vi "CRYInit Data & result stacks global.vi"(8 "Set Value":bool, 9 "No Project Exist?":bool=TRUE, 10 "Pause Proc":bool, 11 "Init?":bool) -> ()   [LabVIEW 2013]
uses:
  CRYData & result stacks global.vi
  CRYWindow/SubVI/CRYMain Sub Window Global.vi
panel:
  # "Set Toolbar Time, Lot, S/N, Iteration value."
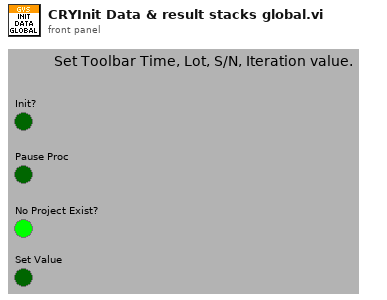
[diagram p1: front panel]
types:
  T1 = enum8{"Enabled", "Disabled", "Disabled and Grayed Out"}
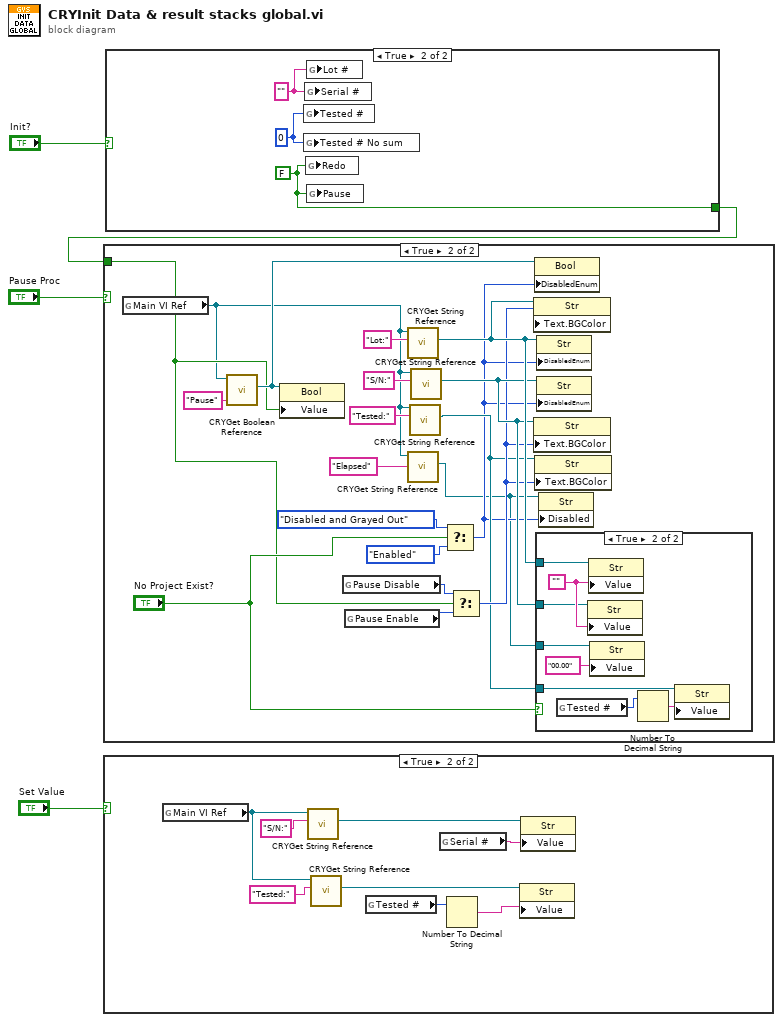
[diagram p0: block diagram]
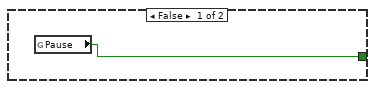
[diagram p3: hidden frame]
diagram:
  n1 = case shown="True" "Set Value" {
    frame False {
    }
    frame True {
      n2 = global read "CRYMain Sub Window Global.vi" "Main VI Ref"() -> (w9:refnum<vi>)
      n3 = call "CRYGet String Reference.vi"("Label Name"="S/N:", "VI Refnum"=w9) -> ("String Ref Out"=w11:refnum<vi>)  [unwired: 7 in, 2 out]
      n4 = call "CRYGet String Reference.vi"("Label Name"="Tested:", "VI Refnum"=w9) -> ("String Ref Out"=w7:refnum<vi>)  [unwired: 7 in, 2 out]
      n5 = global read "CRYData & result stacks global.vi" "Tested #"() -> (w5:u16)
      n6 = global read "CRYData & result stacks global.vi" "Serial #"() -> (w10:string)
      n7 = Number To Decimal String(number=w5) -> (decimal integer string=w6:string)  [unwired: 1 in]
      n8 = property class="Str"(reference=w7, "Value"=w6) -> ()  [unwired: 1 in, 2 out]
      n9 = property class="Str"(reference=w11, "Value"=w10) -> ()  [unwired: 1 in, 2 out]
    }
  }
  n10 = case shown="True" "Init?" {
    tunnel: [w13 w16] -> w2
    frame False {
      n11 = global read "CRYData & result stacks global.vi" "Pause"() -> (w13:bool)
    }
    frame True {
      w14 = u16 0 ("Tested #")
      w15 = "" ("Serial #")
      w16 = FALSE ("Redo")
      n12 = global write "CRYData & result stacks global.vi" "Tested #"(w14) -> ()
      n13 = global write "CRYData & result stacks global.vi" "Tested # No sum"(w14) -> ()
      n14 = global write "CRYData & result stacks global.vi" "Serial #"(w15) -> ()
      n15 = global write "CRYData & result stacks global.vi" "Redo"(w16) -> ()
      n16 = global write "CRYData & result stacks global.vi" "Lot #"(w15) -> ()
      n17 = global write "CRYData & result stacks global.vi" "Pause"(w16) -> ()
    }
  }
  n18 = case shown="True" "Pause Proc" {
    tunnel: w2 -> [_ w24]
    frame False {
    }
    frame True {
      n19 = global read "CRYMain Sub Window Global.vi" "Main VI Ref"() -> (w19:refnum<vi>)
      n20 = call "CRYGet Boolean Reference.vi"("Label Name"="Pause", "VI Refnum"=w19) -> ("Boolean Ref"=w26:refnum<vi>)  [unwired: 9 out]
      n21 = property class="Bool"(reference=w26, "Value"=w24) -> ()  [unwired: 1 in, 2 out]
      n22 = global read "CRYMain Sub Window Global.vi" "Pause Disable"() -> (w31:u32)
      n23 = global read "CRYMain Sub Window Global.vi" "Pause Enable"() -> (w30:u32)
      n24 = call "CRYGet String Reference.vi"("Label Name"="Lot:", "VI Refnum"=w19) -> ("String Ref Out"=w29:refnum<vi>)  [unwired: 7 in, 2 out]
      n25 = call "CRYGet String Reference.vi"("Label Name"="Elapsed", "VI Refnum"=w19) -> ("String Ref Out"=w17:refnum<vi>)  [unwired: 7 in, 2 out]
      n26 = call "CRYGet String Reference.vi"("Label Name"="Tested:", "VI Refnum"=w19) -> ("String Ref Out"=w21:refnum<vi>)  [unwired: 7 in, 2 out]
      n27 = call "CRYGet String Reference.vi"("Label Name"="S/N:", "VI Refnum"=w19) -> ("String Ref Out"=w28:refnum<vi>)  [unwired: 7 in, 2 out]
      n28 = Select(t=T1."Disabled and Grayed Out" ("Disabled"), s="No Project Exist?", f=T1."Enabled" ("Disabled")) -> (s? t:f=w18:T1)
      n29 = Select(t=w31, s=w24, f=w30) -> (s? t:f=w23:u32)
      n30 = property class="Str"(reference=w29, "Text.BGColor"=w23) -> ()  [unwired: 1 in, 2 out]
      n31 = property class="Str"(reference=w28, "Text.BGColor"=w23) -> ()  [unwired: 1 in, 2 out]
      n32 = property class="Bool"(reference=w26, "DisabledEnum"=w18) -> ()  [unwired: 1 in, 2 out]
      n33 = property class="Str"(reference=w21, "Text.BGColor"=w23) -> ()  [unwired: 1 in, 2 out]
      n34 = case shown="True" "No Project Exist?" {
        tunnel: w29 -> [_ w43]
        tunnel: w28 -> [_ w41]
        tunnel: w21 -> [_ w40]
        tunnel: w17 -> [_ w36]
        frame False {
        }
        frame True {
          w42 = "" ("Value")
          n35 = global read "CRYData & result stacks global.vi" "Tested #"() -> (w39:u16)
          n36 = property class="Str"(reference=w41, "Value"=w42) -> ()  [unwired: 1 in, 2 out]
          n37 = property class="Str"(reference=w43, "Value"=w42) -> ()  [unwired: 1 in, 2 out]
          n38 = property class="Str"(reference=w36, "Value"="00.00") -> ()  [unwired: 1 in, 2 out]
          n39 = Number To Decimal String(number=w39) -> (decimal integer string=w38:string)  [unwired: 1 in]
          n40 = property class="Str"(reference=w40, "Value"=w38) -> ()  [unwired: 1 in, 2 out]
        }
      }
      n41 = property class="Str"(reference=w29, "DisabledEnum"=w18) -> ()  [unwired: 1 in, 2 out]
      n42 = property class="Str"(reference=w28, "DisabledEnum"=w18) -> ()  [unwired: 1 in, 2 out]
      n43 = property class="Str"(reference=w17, "Disabled"=w18) -> ()  [unwired: 1 in, 2 out]
    }
  }
